vi "Receive from CS.vi"(8 "error in (no error)":errorcluster, 11 "CS in":refnum<class "CS.lvclass">) -> (0 "error out":errorcluster, 2 "Response string":string, 3 "CS out":refnum<class "CS.lvclass">)   [LabVIEW 2016, in "CS.lvclass"]
uses:
  Lib.llb/CS.lvclass
  Lib.llb/CS.lvclass/CS.ctl
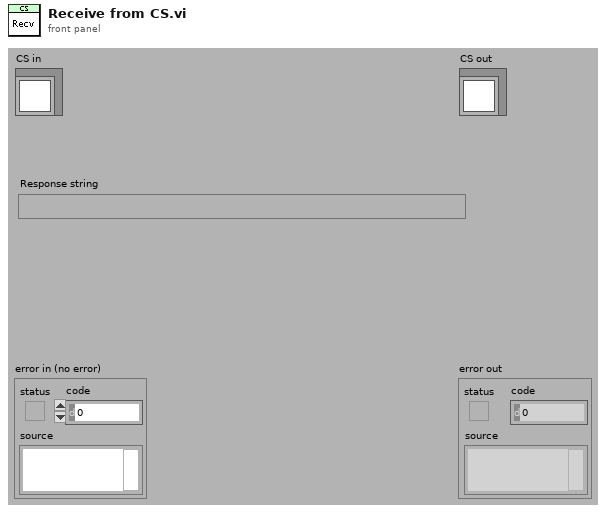
[diagram p1: front panel]
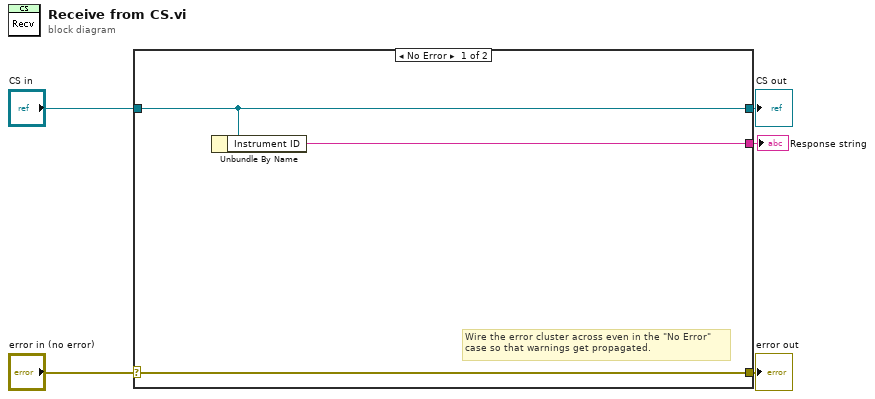
[diagram p0: block diagram]
diagram:
  n1 = case shown="No Error" "error in (no error)" {
    selector: "error in (no error)" -> [w6 w10]
    tunnel: [w6 w10] -> w4
    tunnel: [w7 w9] -> w2
    tunnel: "CS in" -> [w7 w9]
    tunnel: [w8 _] -> w1
    frame No Error {
      # "Wire the error cluster across even in the \"No Error\"\ncase so that warnings get propagated."
      n2 = Unbundle By Name(w7) -> ("Instrument ID"=w8:string)
    }
    frame Error {
    }
  }
  "error out" <- w4
  "CS out" <- w2
  "Response string" <- w1
